vi "CSC_ModCuffLocation.vi"(8 "error in (no error)":errorcluster, 9 "CuffID":i32, 10 "CuffInLCS(xyz)":dbl[](array[numeric]), 11 "CSC in":refnum<class "CableSerialChain.lvclass">) -> (0 "error out":errorcluster, 3 "CSC out":refnum<class "CableSerialChain.lvclass">)   [LabVIEW 2015, in "CableSerialChain.lvclass"]
uses:
  CableSerialChain.lvclass
  CableSerialChain.lvclass/CableSerialChain.ctl
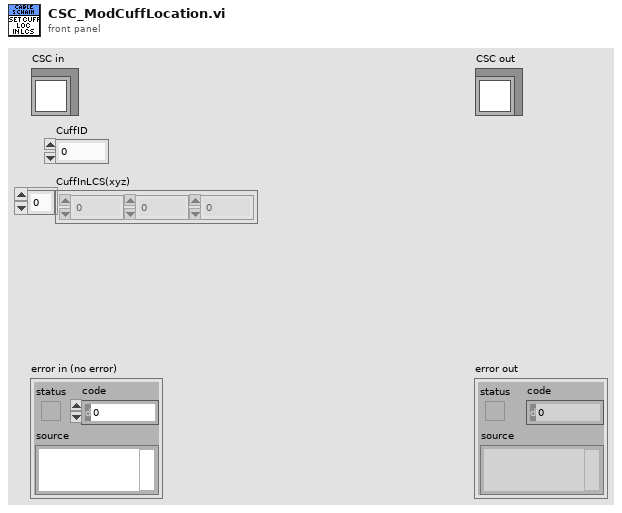
[diagram p1: front panel]
types:
  T1 = typedef "CableSerialChain.lvclass/Cuff.ctl" = cluster{"BodyID":i32, "CoM(CuffCS)":T2, "Mass(kg)":dbl, "CablePts(CuffCS)":T2[], "Cuff->Body":T3}
  T2 = typedef "Bodies.lvclass/PointOnBody.ctl" = cluster{"Coord4":dbl[], "ID":i32}
  T3 = typedef "NI_Matrix.lvlib/RealMatrix.ctl" = dbl[][]
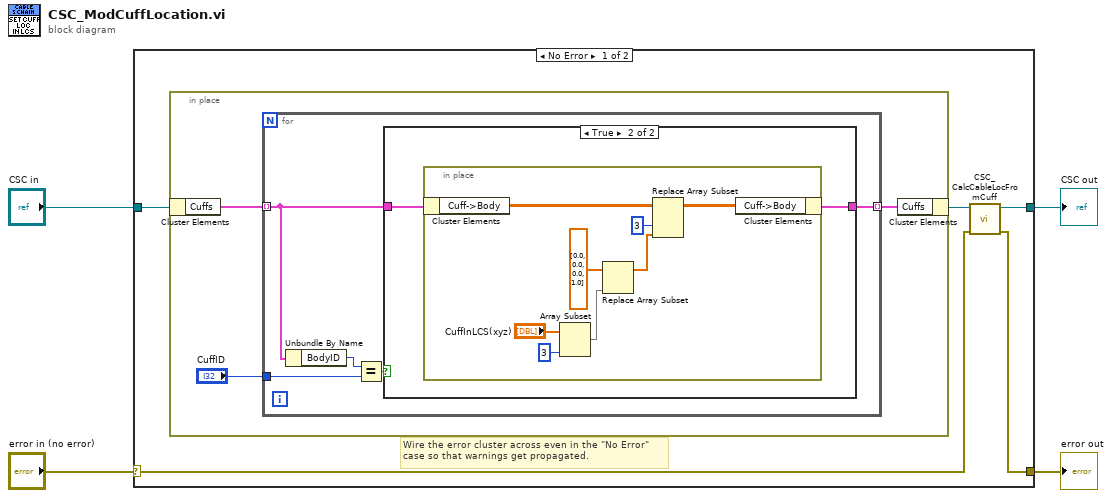
[diagram p0: block diagram]
diagram:
  n1 = case shown="No Error" "error in (no error)" {
    selector: "error in (no error)" -> [w6 w30]
    tunnel: [w5 w30] -> w3
    tunnel: "CSC in" -> [w9 w29]
    tunnel: [w7 w29] -> w1
    frame No Error {
      # "Wire the error cluster across even in the \"No Error\"\ncase so that warnings get propagated."
      n2 = in-place {
        n3 = in-place-cluster #1(w9) -> ("Cuffs"=w12:T1[])
        n4 = for {
          tunnel: w12 -> [w14] mode=indexing
          tunnel: "CuffID" -> [w16]
          tunnel: [w13] -> w10 mode=indexing
          n5 = Unbundle By Name(w14) -> ("BodyID"=w17:i32)
          n6 = Equal?(x=w17, y=w16) -> (x = y?=w15:bool)
          n7 = case shown="True" w15 {
            tunnel: w14 -> [w18 w20]
            tunnel: [w18 w19] -> w13
            frame False {
            }
            frame True {
              n8 = in-place {
                n9 = in-place-cluster #2(w20) -> ("Cuff->Body"=w28:T3)
                n10 = Array Subset(array="CuffInLCS(xyz)", length=3) -> (w21:dbl[])  [unwired: 1 in]
                n11 = Replace Array Subset(array=dbl[] [0.0, 0.0, 0.0, 1.0], new element=w21) -> (w24:dbl[])  [unwired: 1 in]
                n12 = Replace Array Subset(array=w28, new element=w24, index (col)=3 ("disabled index (col)")) -> (w27:T3)  [unwired: 1 in]
                n13 = in-place-cluster #2("Cuff->Body"=w27) -> (w19:T1)
              }
            }
          }
        }
        n14 = in-place-cluster #1("Cuffs"=w10) -> (w8:refnum<class "CableSerialChain.lvclass">)
      }
      n15 = call "CSC_CalcCableLocFromCuff.vi"("error in (no error)"=w6, "C-Alex"=w8) -> ("error out"=w5:errorcluster, "C-Alex Out"=w7:refnum<class "CableSerialChain.lvclass">)  [unwired: 8 in]
    }
    frame Error {
    }
  }
  "error out" <- w3
  "CSC out" <- w1
